vi "Test Result Event to JSON.vi"(9 "indent level":i32, 10 "Test Results Event":T1[](array[typedef])) -> (2 "<JSON>Test Results Event":string)   [LabVIEW 2013, in "Caraya.lvlib" / "Test Result.lvclass"]
uses:
  Test Result.lvclass
  Node Results.ctl
  Test Node.ctl
  Test Registration Data.ctl
  Assert Event Data.ctl
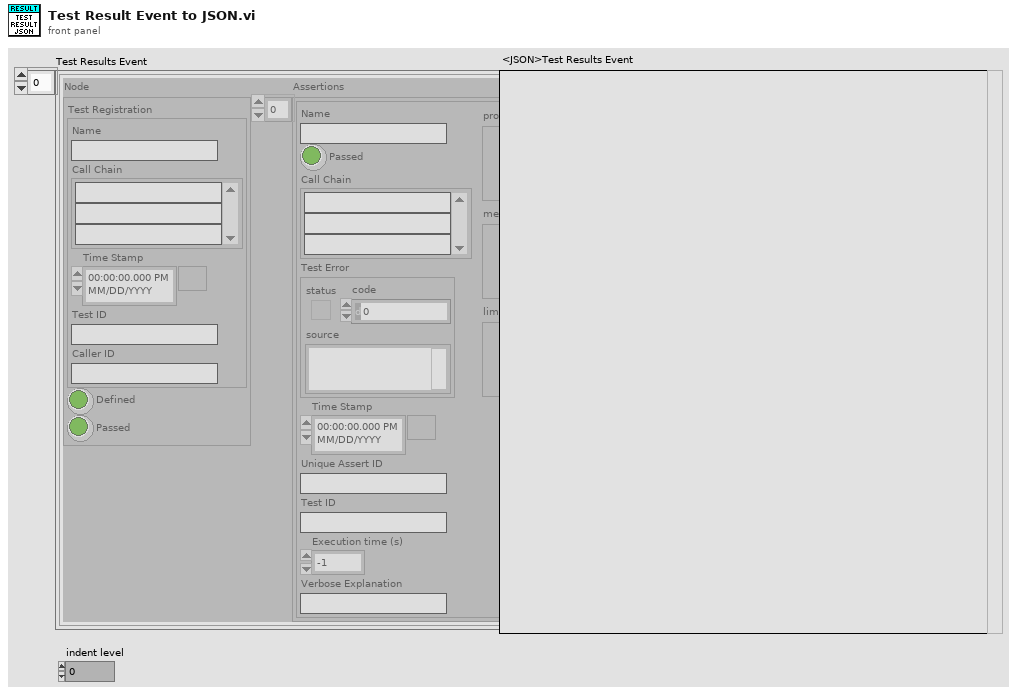
[diagram p1: front panel]
types:
  T1 = typedef "Caraya.lvlib/Test Result.lvclass/Node Results.ctl" = cluster{"Node":T2, "Assertions":T4[]}
  T2 = typedef "Caraya.lvlib/Test Result.lvclass/Test Node.ctl" = cluster{"Test Registration":T3, "Defined":bool, "Passed":bool}
  T3 = typedef "Caraya.lvlib/Test Result.lvclass/Test Registration Data.ctl" = cluster{"Name":string, "Call Chain":string[], "Time Stamp":timestamp, "Test ID":string, "Caller ID":string}
  T4 = typedef "Caraya.lvlib/Test Result.lvclass/Assert Event Data.ctl" = cluster{"Name":string, "Passed":bool, "Call Chain":string[], "Test Error":errorcluster, "Time Stamp":timestamp, "Unique Assert ID":string, "Test ID":string, "Execution time (s)":dbl, "Verbose Explanation":string, "properties":variant, "measurements":variant, "limits":variant}
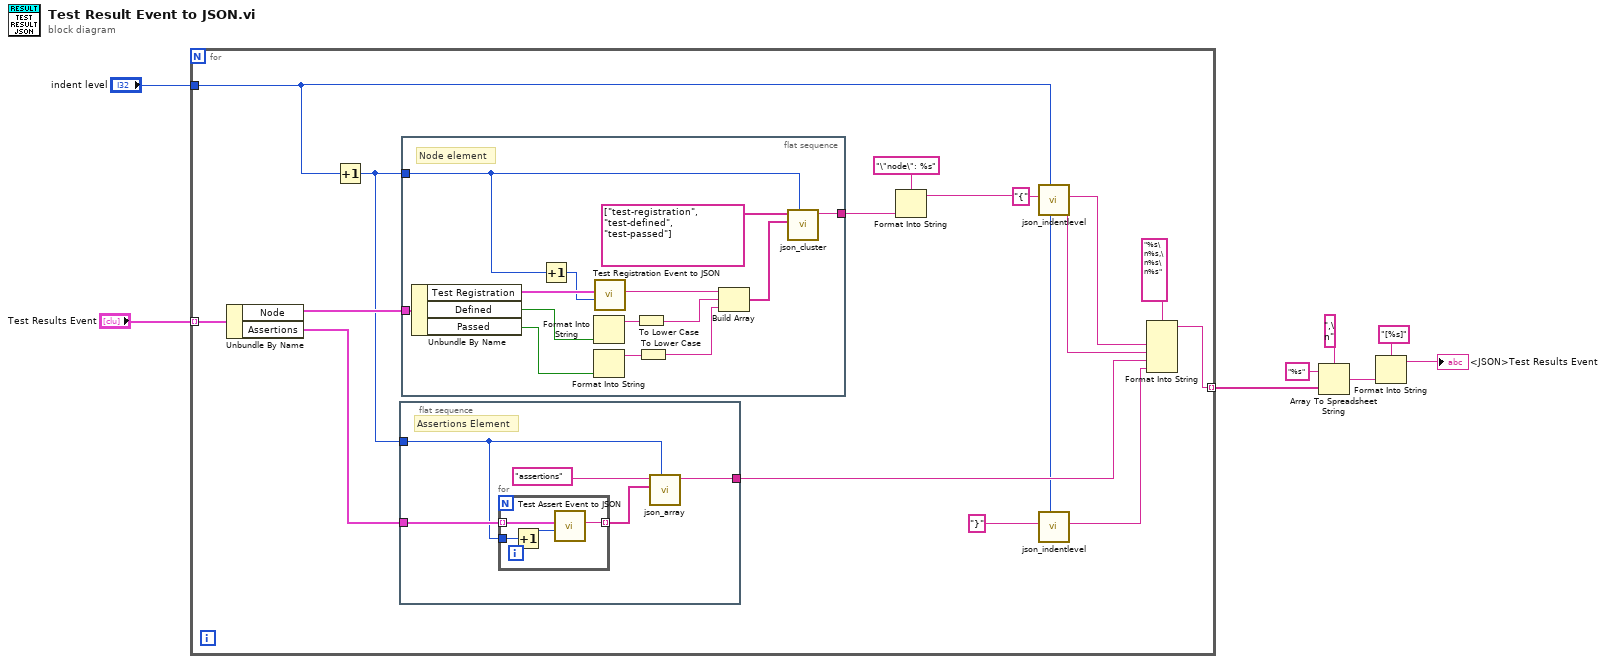
[diagram p0: block diagram]
diagram:
  n1 = for {
    tunnel: "Test Results Event" -> [w22] mode=indexing
    tunnel: [w20] -> w5 mode=indexing
    tunnel: "indent level" -> [w9]
    n2 = Unbundle By Name(w22) -> ("Node"=w23:T2, "Assertions"=w18:T4[])
    n3 = Increment(x=w9) -> (x+1=w10:i32)
    n4 = flat-sequence {
      tunnel: [w28] -> w19
      tunnel: w18 -> [w27]
      tunnel: w10 -> [w24]
      frame #0 {
        # "Assertions Element"
        n5 = for {
          tunnel: w27 -> [w32] mode=indexing
          tunnel: [w31] -> w25 mode=indexing
          tunnel: w24 -> [w30]
          n6 = Increment(x=w30) -> (x+1=w29:i32)
          n7 = call "Test Assert Event to JSON.vi"("indent level"=w29, "Test Event"=w32) -> ("<JSON>Assertion Event"=w31:string)  [unwired: 9 in]
        }
        n8 = call "json_array.vi"("indent level"=w24, "Array of JSON Elements"=w25, "name"="assertions" ("string")) -> ("indented string"=w28:string)  [unwired: 8 in]
      }
    }
    n9 = flat-sequence {
      tunnel: w23 -> [w46]
      tunnel: [w39] -> w12
      tunnel: w10 -> [w33]
      frame #0 {
        # "Node element"
        n10 = Unbundle By Name(w46) -> ("Test Registration"=w45:T3, "Defined"=w43:bool, "Passed"=w41:bool)
        n11 = Increment(x=w33) -> (x+1=w40:i32)
        n12 = Format Into String(w43) -> (resulting string=w44:string)  [unwired: 3 in, 1 out]
        n13 = Format Into String(w41) -> (resulting string=w42:string)  [unwired: 3 in, 1 out]
        n14 = call "Test Registration Event to JSON.vi"("indent level"=w40, "Test Registration"=w45) -> ("<JSON>Test Registration Event"=w38:string)  [unwired: 9 in]
        n15 = To Lower Case(string=w44) -> (all lower case string=w37:string)
        n16 = To Lower Case(string=w42) -> (all lower case string=w36:string)
        n17 = Build Array(w38, w37, w36) -> (w34:string[])
        n18 = call "json_cluster.vi"("indent level"=w33, "array of JSON values"=w34, "array of element names"=string[] ["test-registration", "test-defined", "test-passed"] ("appended array")) -> ("indented string"=w39:string)  [unwired: 8 in]
      }
    }
    n19 = Format Into String(format string="\"node\": %s" ("string"), w12) -> (resulting string=w11:string)  [unwired: 2 in, 1 out]
    n20 = call "json_indentlevel.vi"("indent level"=w9, "string"="{") -> ("indented string"=w16:string)  [unwired: 9 in]
    n21 = call "json_indentlevel.vi"("indent level"=w9, "string"="}") -> ("indented string"=w14:string)  [unwired: 9 in]
    n22 = Format Into String(format string="%s\n%s,\n%s\n%s" ("delimiter (Tab)"), w16, w11, w19, w14) -> (resulting string=w20:string)  [unwired: 2 in, 1 out]
  }
  n23 = Array To Spreadsheet String(delimiter (Tab)=",\n", array=w5, 3:"%s" ("format string")) -> (spreadsheet string=w3:string)
  n24 = Format Into String(format string="[%s]" ("delimiter (Tab)"), w3) -> (resulting string=→"<JSON>Test Results Event":string)  [unwired: 2 in, 1 out]
